vi "Demo.vi"() -> ()   [LabVIEW 2021, in "CollapsePanel.lvclass"]
uses:
  CollapsePanel.lvclass
  SubVIs/collapse direction.ctl
  CollapsePanel.lvclass/CollapsePanel.ctl
  SubVIs/splitter position calc.vi
panel:
  in  "OK Button 4":bool
  in  "OK Button 2":bool
  in  "Up":bool
  in  "Left":bool
  in  "Right":bool
  in  "Down":bool
  in  "OK Button 3":bool
  in  "OK Button":bool
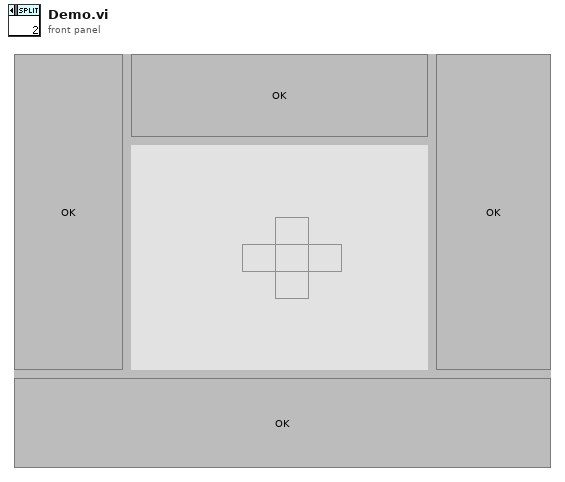
[diagram p1: front panel]
types:
  T1 = typedef "CollapsePanel.lvclass/collapse direction.ctl" = enum16{"Left", "Right", "Up", "Down"}
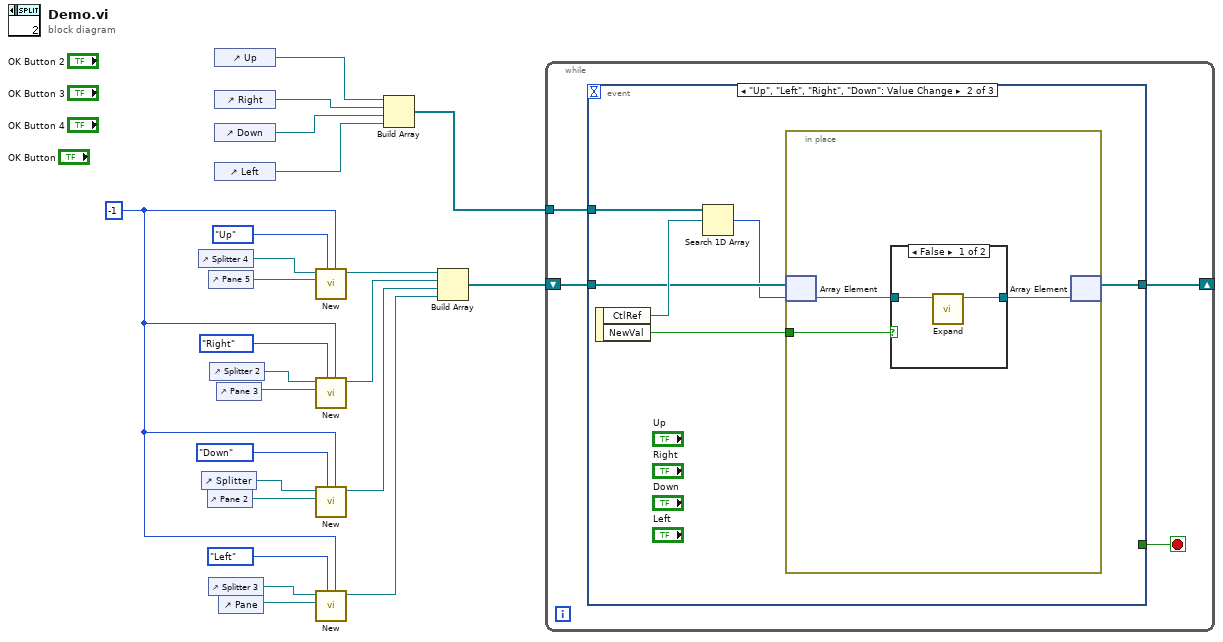
[diagram p0: block diagram]
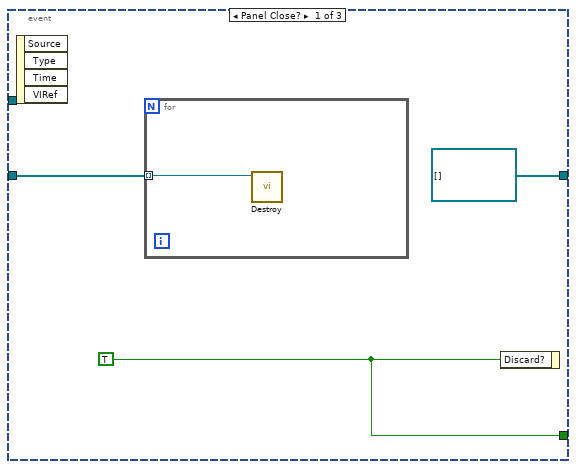
[diagram p2: hidden frame]
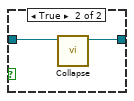
[diagram p3: hidden frame]
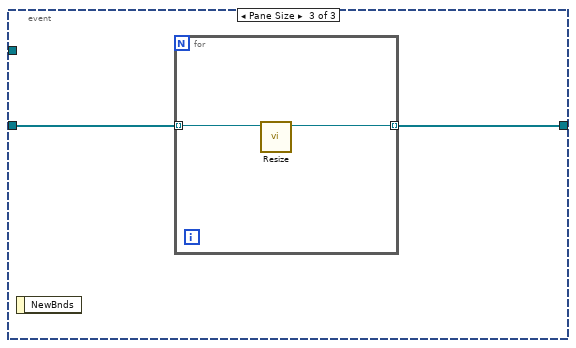
[diagram p4: hidden frame]
diagram:
  w1 = -1 ("ExpandSize")
  n1 = control-ref of="Splitter 4"() -> (w23:refnum<vi>)
  n2 = control-ref of="Splitter"() -> (w14:refnum<vi>)
  n3 = control-ref of="Pane 2"() -> (w15:refnum<vi>)
  n4 = control-ref of="Pane 5"() -> (w22:refnum<vi>)
  n5 = control-ref of="Splitter 3"() -> (w12:refnum<vi>)
  n6 = control-ref of="Splitter 2"() -> (w16:refnum<vi>)
  n7 = control-ref of="Up"() -> (w5:refnum<vi>)
  n8 = control-ref of="Right"() -> (w3:refnum<vi>)
  n9 = control-ref of="Down"() -> (w2:refnum<vi>)
  n10 = control-ref of="Left"() -> (w6:refnum<vi>)
  n11 = control-ref of="Pane 3"() -> (w17:refnum<vi>)
  n12 = control-ref of="Pane"() -> (w13:refnum<vi>)
  n13 = call "New.vi"("ExpandSize (starting size)"=w1, "CollapseDirection"=collapse_direction."Up", "Pane"=w22, "Splitter"=w23) -> ("CollapsePanel out"=w11:refnum<class "CollapsePanel.lvclass">)  [unwired: 6 in, 1 out]
  n14 = call "New.vi"("ExpandSize (starting size)"=w1, "CollapseDirection"=collapse_direction."Right", "Pane"=w17, "Splitter"=w16) -> ("CollapsePanel out"=w10:refnum<class "CollapsePanel.lvclass">)  [unwired: 6 in, 1 out]
  n15 = call "New.vi"("ExpandSize (starting size)"=w1, "CollapseDirection"=collapse_direction."Down", "Pane"=w15, "Splitter"=w14) -> ("CollapsePanel out"=w9:refnum<class "CollapsePanel.lvclass">)  [unwired: 6 in, 1 out]
  n16 = call "New.vi"("ExpandSize (starting size)"=w1, "CollapseDirection"=collapse_direction."Left", "Pane"=w13, "Splitter"=w12) -> ("CollapsePanel out"=w8:refnum<class "CollapsePanel.lvclass">)  [unwired: 6 in, 1 out]
  n17 = Build Array(w5, w3, w2, w6) -> (w4:refnum<vi>[])
  n18 = Build Array(w11, w10, w9, w8) -> (w7:refnum<class "CollapsePanel.lvclass">[])
  n19 = while {
    tunnel: w4 -> [w25]
    shift-right: [w24] -> _
    shift-left: w7 -> [w26]
    stop <- w27 stop-if-true
    n20 = event shown="[1] \"Up\", \"Left\", \"Right\", \"Down\": Value Change" {
      selector: _ -> [_ _ _]
      dyn-events: _ -> [_ _ _]
      timeout: _ -> [_ _ _]
      tunnel: [w30 _ _] -> w27
      tunnel: w26 -> [w29 w34 w46]
      tunnel: w25 -> [_ w36 _]
      tunnel: [refnum<class "CollapsePanel.lvclass">[] [] w32 w45] -> w24
      event Panel Close? {
        w30 = TRUE ("Discard?")
        n21 = event-data() -> ()  [unwired: 1 in, 4 out]
        n22 = for {
          tunnel: w29 -> [w31] mode=indexing
          n23 = call "Destroy.vi"("CollapsePanel in"=w31) -> ()  [unwired: 10 in, 1 out]
        }
        n24 = event-data("Discard?"=w30) -> ()  [unwired: 1 in, 1 out]
      }
      event "Up", "Left", "Right", "Down": Value Change {
        n25 = event-data() -> ("CtlRef"=w35:refnum<vi>, "NewVal"=w37:bool)  [unwired: 1 in]
        n26 = Search 1D Array(1D array=w36, element=w35) -> (index of element=w33:i32)  [unwired: 1 in]
        n27 = in-place {
          in-place-border: w37 -> [w40]
          n28 = in-place-array #1(w34, w33) -> (w39:refnum<class "CollapsePanel.lvclass">)
          n29 = case shown="False" w40 {
            tunnel: w39 -> [w42 w44]
            tunnel: [w41 w43] -> w38
            frame False {
              n30 = call "Expand.vi"("CollapsePanel in"=w42) -> ("CollapsePanel out"=w41:refnum<class "CollapsePanel.lvclass">)  [unwired: 9 in, 1 out]
            }
            frame True {
              n31 = call "Collapse.vi"("CollapsePanel in"=w44) -> ("CollapsePanel out"=w43:refnum<class "CollapsePanel.lvclass">)  [unwired: 9 in, 1 out]
            }
          }
          n32 = in-place-array #1(w38) -> (w32:refnum<class "CollapsePanel.lvclass">[])  [unwired: 1 out]
        }
      }
      event Pane Size {
        n33 = event-data() -> ()  [unwired: 1 in, 1 out]
        n34 = for {
          tunnel: w46 -> [w48] mode=indexing
          tunnel: [w47] -> w45 mode=indexing
          n35 = call "Resize.vi"("CollapsePanel in"=w48) -> ("CollapsePanel out"=w47:refnum<class "CollapsePanel.lvclass">)  [unwired: 9 in, 1 out]
        }
      }
    }
  }
